vi "Prober_MoveToXYZTheta.vi"(6 "Theta location [mdeg]":string="none", 7 "AlessiRel6100 in":refnum<class "AlessiRel6100.lvclass">, 8 "error in (no error)":errorcluster, 9 "Z location [µm]":string="none", 10 "Y location [µm]":string="none", 11 "X location [µm]":string="none") -> (0 "error out":errorcluster, 2 "String":string, 3 "AlessiRel6100 out":refnum<class "AlessiRel6100.lvclass">)   [LabVIEW 2019, in "AlessiRel6100.lvclass"]
uses:
  AlessiRel6100.lvclass
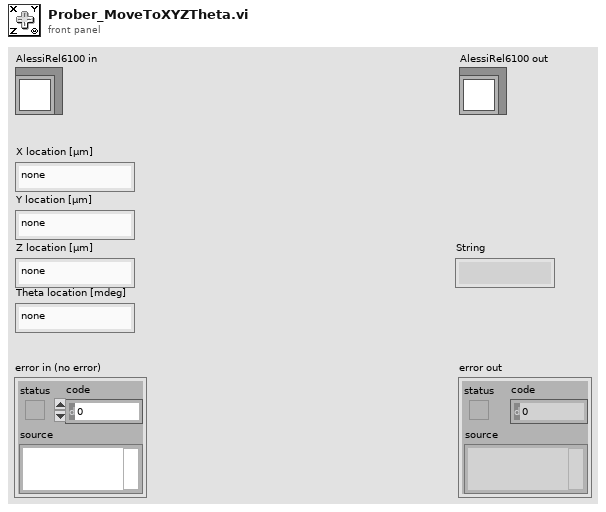
[diagram p1: front panel]
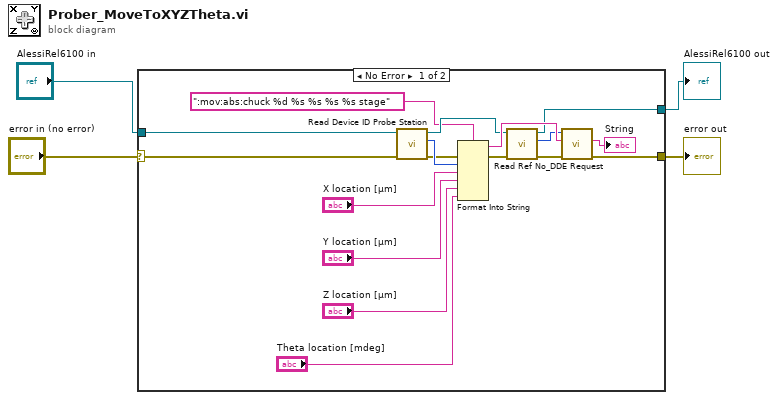
[diagram p0: block diagram]
diagram:
  n1 = case shown="No Error" "error in (no error)" {
    selector: "error in (no error)" -> [w13 w23]
    tunnel: "AlessiRel6100 in" -> [w12 w22]
    tunnel: [w11 w22] -> w2
    tunnel: [w10 w23] -> w1
    frame No Error {
      n2 = call-dynamic "Read Device ID Probe Station.vi"("error in (no error)"=w13, "AlessiRel6100 in"=w12) -> ("error out"=w18:errorcluster, "Device ID Probe Station"=w20:u32, "AlessiRel6100 out"=w19:refnum<class "AlessiRel6100.lvclass">)  [unwired: 7 in]
      n3 = Format Into String(format string=":mov:abs:chuck %d %s %s %s %s stage", error in=w18, w20, "X location [µm]", "Y location [µm]", "Z location [µm]", "Theta location [mdeg]") -> (resulting string=w21:string, error out=w16:errorcluster)  [unwired: 1 in]
      n4 = call-dynamic "Read Ref No_.vi"("error in (no error)"=w16, "AlessiRel6100 in"=w19) -> ("error out"=w15:errorcluster, "Ref No."=w14:u32, "AlessiRel6100 out"=w11:refnum<class "AlessiRel6100.lvclass">)  [unwired: 7 in]
      n5 = call <vilib>:"DDE Request.vi"("error in (no error)"=w15, "item"=w21, "conversation refnum in"=w14) -> ("error out"=w10:errorcluster, "data"=→"String":string)  [unwired: 4 in, 1 out]
    }
    frame Error {
    }
  }
  "error out" <- w1
  "AlessiRel6100 out" <- w2
